vi "parseDataPacket.vi"(8 "error in (no error)":errorcluster, 11 "data in":string) -> (0 "error out":errorcluster, 3 "DataPacket":T1)   [LabVIEW 2016]
uses:
  Controls/visionData.ctl
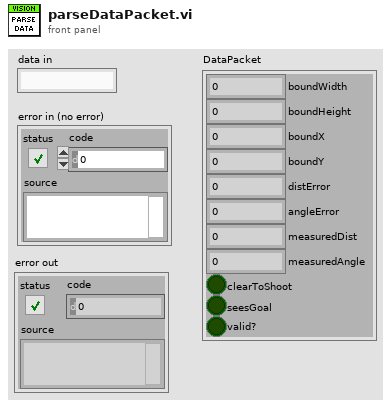
[diagram p1: front panel]
types:
  T1 = typedef "visionData.ctl" = cluster{"boundWidth":dbl, "boundHeight":dbl, "boundX":dbl, "boundY":dbl, "distError":dbl, "angleError":dbl, "measuredDist":dbl, "measuredAngle":dbl, "clearToShoot":bool, "seesGoal":bool, "valid?":bool}
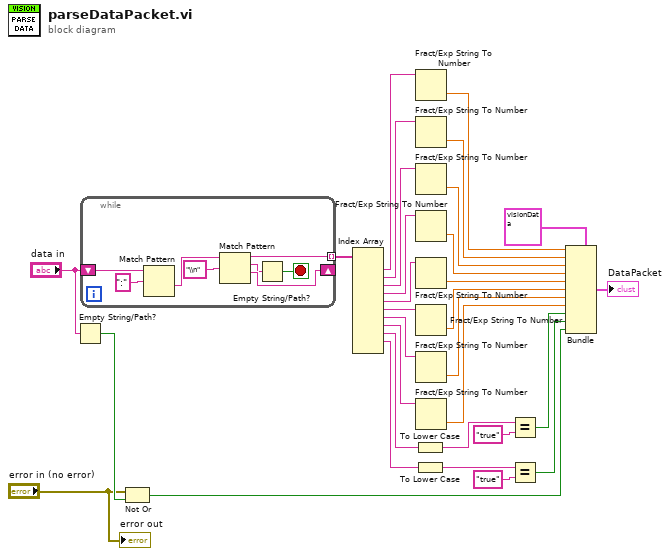
[diagram p0: block diagram]
diagram:
  n1 = Empty String/Path?(string/path="data in") -> (empty?=w29:bool)
  n2 = while {
    shift-right: [w35] -> _
    shift-left: "data in" -> [w39]
    tunnel: [w32] -> w5 mode=indexing
    stop <- w33 stop-if-true
    n3 = Match Pattern(string=w39, regular expression=":") -> (after substring=w37:string)  [unwired: 1 in, 3 out]
    n4 = Match Pattern(string=w37, regular expression="\\n") -> (before substring=w32:string, match substring=w34:string, after substring=w35:string)  [unwired: 1 in, 1 out]
    n5 = Empty String/Path?(string/path=w34) -> (empty?=w33:bool)
  }
  n6 = Not Or(1:w29, 2:"error in (no error)") -> (0:w30:bool)
  n7 = Index Array(array=w5) -> (element #1=w7:string, element #2=w2:string, element #3=w8:string, element #4=w9:string, element #5=w12:string, element #6=w13:string, element #7=w14:string, element #8=w15:string, element #9=w20:string, element #10=w26:string)  [unwired: 11 in, 1 out]
  n8 = To Lower Case(string=w20) -> (all lower case string=w21:string)
  n9 = To Lower Case(string=w26) -> (all lower case string=w25:string)
  n10 = Fract/Exp String To Number(string=w7) -> (number=w3:dbl)  [unwired: 3 in, 1 out]
  n11 = Fract/Exp String To Number(string=w2) -> (number=w4:dbl)  [unwired: 3 in, 1 out]
  n12 = Fract/Exp String To Number(string=w8) -> (number=w10:dbl)  [unwired: 3 in, 1 out]
  n13 = Fract/Exp String To Number(string=w9) -> (number=w11:dbl)  [unwired: 3 in, 1 out]
  n14 = Fract/Exp String To Number(string=w12) -> (number=w16:dbl)  [unwired: 3 in, 1 out]
  n15 = Fract/Exp String To Number(string=w13) -> (number=w17:dbl)  [unwired: 3 in, 1 out]
  n16 = Fract/Exp String To Number(string=w14) -> (number=w18:dbl)  [unwired: 3 in, 1 out]
  n17 = Fract/Exp String To Number(string=w15) -> (number=w19:dbl)  [unwired: 3 in, 1 out]
  n18 = Equal?(x=w21, y="true") -> (x = y?=w23:bool)
  n19 = Equal?(x=w25, y="true") -> (x = y?=w27:bool)
  n20 = Bundle(cluster=T1 {"boundWidth"=0.0, "boundHeight"=0.0, "boundX"=0.0, "boundY"=0.0, "distError"=0.0, "angleError"=0.0, "measuredDist"=0.0, "measuredAngle"=0.0, "clearToShoot"=FALSE, "seesGoal"=FALSE, "valid?"=FALSE} ("DataPacket"), "boundWidth"=w3, "boundHeight"=w4, "boundX"=w10, "boundY"=w11, "distError"=w16, "angleError"=w17, "measuredDist"=w18, "measuredAngle"=w19, "clearToShoot"=w23, "seesGoal"=w27, "valid?"=w30) -> (→"DataPacket":T1)
  "error out" <- "error in (no error)"
